vi "meth.SetTableArray.vi"(0 "class.GLue in":refnum<class "class.GLue.lvclass">, 7 "Array":variant, 11 "error in (no error)":errorcluster, 13 "Name":string) -> (4 "class.GLue out":refnum<class "class.GLue.lvclass">, 15 "error out":errorcluster)   [LabVIEW 2014, in "GLue.lvlib" / "class.GLue.lvclass"]
uses:
  class.GLue.lvclass
  class.GLue.lvclass/class.GLue.ctl
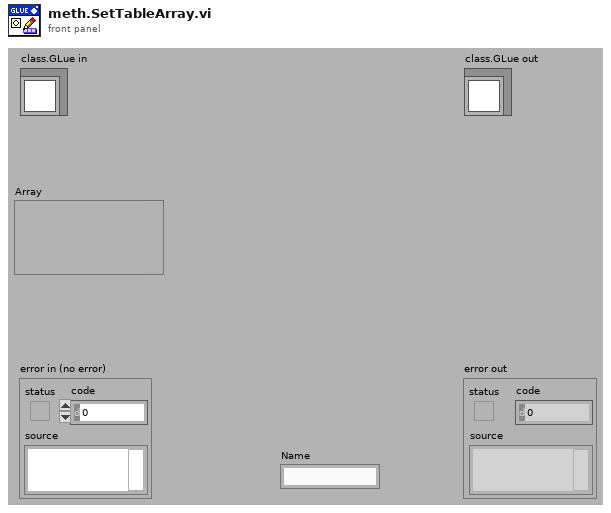
[diagram p1: front panel]
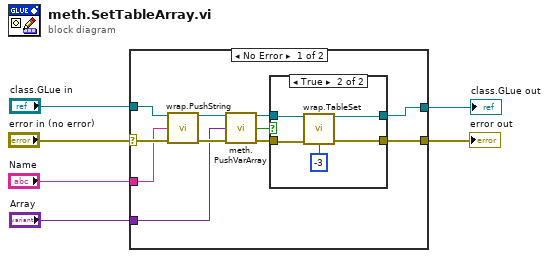
[diagram p0: block diagram]
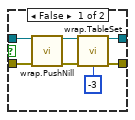
[diagram p2: hidden frame]
diagram:
  n1 = case shown="No Error" "error in (no error)" {
    selector: "error in (no error)" -> [w17 w31]
    tunnel: [w8 w31] -> w5
    tunnel: [w7 w30] -> w3
    tunnel: "class.GLue in" -> [w16 w30]
    tunnel: "Array" -> [w12 _]
    tunnel: "Name" -> [w15 _]
    frame No Error {
      n2 = call "wrap.PushString.vi"("class.GLue in"=w16, "String"=w15, "error in (no error)"=w17) -> ("class.GLue out"=w13:refnum<class "class.GLue.lvclass">, "error out"=w14:errorcluster)  [unwired: 11 in]
      n3 = call "meth.PushVarArray.vi"("class.GLue in"=w13, "VarArray"=w12, "error in (no error)"=w14) -> ("class.GLue out"=w10:refnum<class "class.GLue.lvclass">, "Pushed?"=w11:bool, "error out"=w9:errorcluster)  [unwired: 10 in]
      n4 = case shown="True" w11 {
        tunnel: w10 -> [w24 w28]
        tunnel: w9 -> [w23 w29]
        tunnel: [w19 w25] -> w8
        tunnel: [w18 w26] -> w7
        frame False {
          n5 = call "wrap.PushNill.vi"("class.GLue in"=w24, "error in (no error)"=w23) -> ("class.GLue out"=w20:refnum<class "class.GLue.lvclass">, "error out"=w21:errorcluster)  [unwired: 12 in]
          n6 = call "wrap.TableSet.vi"("class.GLue in"=w20, "error in (no error)"=w21, "Index"=-3) -> ("class.GLue out"=w18:refnum<class "class.GLue.lvclass">, "error out"=w19:errorcluster)  [unwired: 11 in]
        }
        frame True {
          n7 = call "wrap.TableSet.vi"("class.GLue in"=w28, "error in (no error)"=w29, "Index"=-3) -> ("class.GLue out"=w26:refnum<class "class.GLue.lvclass">, "error out"=w25:errorcluster)  [unwired: 11 in]
        }
      }
    }
    frame Error {
    }
  }
  "error out" <- w5
  "class.GLue out" <- w3
